vi "2_venv.vi"() -> ()   [LabVIEW 2024]
uses:
  <vilib>/Python/Open Venv Python Session.vi
panel:
  in  "stop":bool
  in  "input string":string
  out "result":string
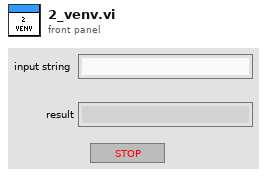
[diagram p1: front panel]
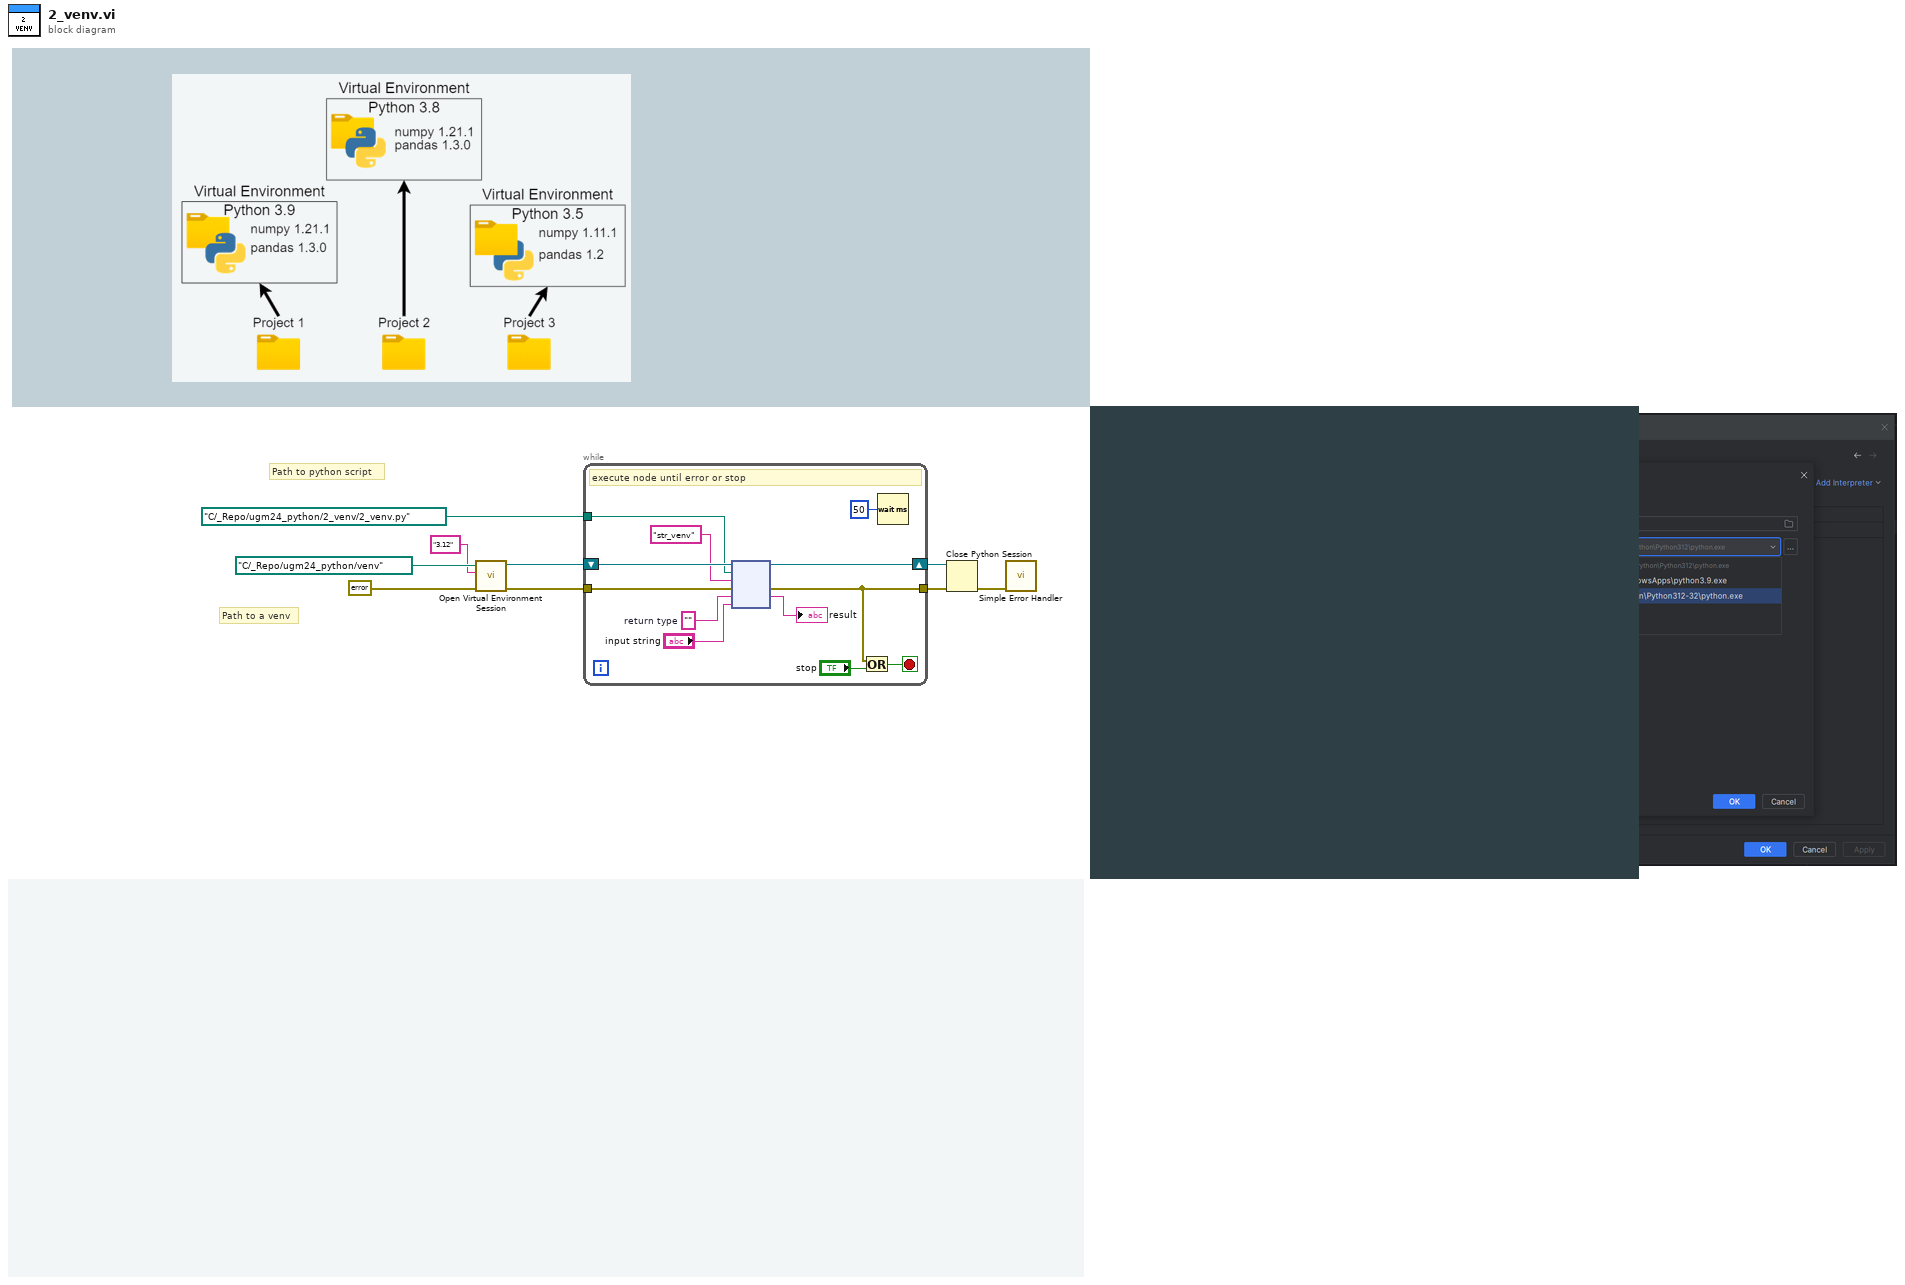
[diagram p0: block diagram]
diagram:
  # "Path to a venv"
  # "Path to python script"
  n1 = call-poly <vilib>:"Open Virtual Environment Session.vi"("error in (no error)"=errorcluster {"status"=FALSE, "code"=0, "source"=""}, "Python version"="3.12", "Env path"=path "C:/_Repo/ugm24_python/venv") -> ("error out"=w4:errorcluster, "session out"=w3:refnum<k35>)  [unwired: 7 in]
  n2 = while {
    tunnel: w4 -> [w21]
    tunnel: path "C:/_Repo/ugm24_python/2_venv/2_venv.py" ("Path") -> [w19]
    tunnel: [w13] -> w8
    shift-right: [w12] -> w7
    shift-left: w3 -> [w20]
    stop <- w15 stop-if-true
    w10 = ""  # return type
    # "execute node until error or stop"
    n3 = node(w20, w19, "str_venv" ("function name"), w21, w10, "input string") -> (w12:refnum<k35>, w13:errorcluster, →"result":string)  [unwired: 1 in, 2 out]
    n4 = Or(x=w13, y="stop") -> (x .or. y?=w15:bool)
    n5 = Wait (ms)(milliseconds to wait=u32 50) -> ()  [unwired: 1 out]
  }
  n6 = Close Python Session(session in=w7, error in=w8) -> (11:w6:errorcluster)
  n7 = call <vilib>:"Simple Error Handler.vi"("error in (no error)"=w6) -> ()  [unwired: 4 in, 5 out]
